vi "Dashboard Main.vi"() -> ()   [LabVIEW 2020]
uses:
  <vilib>/Utility/miscctls.llb/LVRowAndColumnTypeDef.ctl
  <vilib>/event_ctls.llb/eventvkey.ctl
  <vilib>/Rock Robotics/Network Tables/NT Read Boolean.vi
  <vilib>/Rock Robotics/WPI/Dashboard/WPI_DashboardLogging Global.vi
panel:
  in  "Camera Settings Right":T1={"Frame Rate"=30, "Compression"=30, "Size"=1, "DB Camera Config"=FALSE} {"Frame Rate" scale=1.0..30.0; "Compression" scale=100.0..-1.0; "Size" items=["640x480", "320x240", "160x120"]}
  in  "Camera Name Right":string(combo)="No Camera Selection"
  out "Camera Perf":string
  in  "Camera Settings":T1={"Frame Rate"=30, "Compression"=30, "Size"=1, "DB Camera Config"=FALSE} {"Frame Rate" scale=1.0..30.0; "Compression" scale=100.0..-1.0; "Size" items=["640x480", "320x240", "160x120"]}
  in  "TCP":refnum<k5>
  in  "Rec Mode":enum32{"Stop", "Record", "Playback"}(radio)
  out "Robot IP":string
  out "Image Message":string="Timeout in Camera Communications"
  in  "Dashboard Tab":T2(tab)
  out "Hall Effect Low":bool
  out "Limit Switch Stop":bool
  out "Elevator Encoder R":dbl
  out "Elevator Encoder L":dbl
  out "Range Detector":dbl format="%#.0f"
  out "Backwards Drive\nOn":bool
  out "Slow Speed\nOn":bool
  in  "Select Auto":string(combo)="Select Autonomous ..."
  out "NT Connection":bool
  out "Gyro":dbl(knob) scale=0.0..360.0
  out "Mode":T3(ring)=enum."Auto Disabled"
  out "Right Camera Perf":cluster{"Bandwidth (Mbps)":dbl, "FPS":dbl}
  out "Camera Image Right":T4(plugin-control)
  in  "DB/String 9":string
  in  "DB/String 8":string
  in  "DB/String 7":string
  in  "DB/String 6":string
  in  "DB/String 5":string
  in  "DB/String 4":string
  in  "DB/String 3":string
  in  "DB/String 2":string
  in  "DB/String 1":string
  in  "DB/String 0":string
  in  "DB/Slider 0":dbl(slide) scale=0.0..5.0
  in  "DB/Slider 1":dbl(slide) scale=0.0..5.0
  in  "DB/Slider 2":dbl(slide) scale=0.0..5.0
  in  "DB/Slider 3":dbl(slide) scale=0.0..5.0
  out "DB/LED 3":bool
  out "DB/LED 2":bool
  out "DB/LED 1":bool
  out "DB/LED 0":bool
  in  "DB/Button 3":bool
  in  "DB/Button 2":bool
  in  "DB/Button 1":bool
  in  "DB/Button 0":bool caption="New Name"
  in  "Test Slider":dbl(slide) scale=0.0..100.0 scale format="%#_3g"
  in  "On/Off":bool caption="Solenoid"
  in  "Test Name":u16(ring) items=["Select the test to run..."]
  in  "Test Tree":string(tree)
  in  "Motor":cluster{"Value":dbl, "Enable":bool} {"Value" scale=-1.0..1.0 scale format="%#_3g"}
  out "Progress":T5 {"Test Progress" scale=0.0..100.0}
  in  "Rev/Fwd":cluster{"Forward":bool, "Reverse":bool}
  in  "Test Ring":u16(ring) items=["Monochrome", "Color"]
  out "Cmd Status":string
  in  "Execute Command":bool
  in  "Command Params":string[][](table)
  in  "Command Selection":i32(listbox)
  in  "CheckList":i32(listbox)
  out "Tree":string(tree)
  out "Camera Image":T4(plugin-control)
  out "Background":bool
  in  "Camera Name":string(combo)="No Camera Selection"
  # "HW"
  # "HW"
  # "This tab is a great place for autonomous settings and robot-specific values.\nPlace controls and indicators inside this tab and match name to\nDashboard Variables on robot. You can also delete this comment."
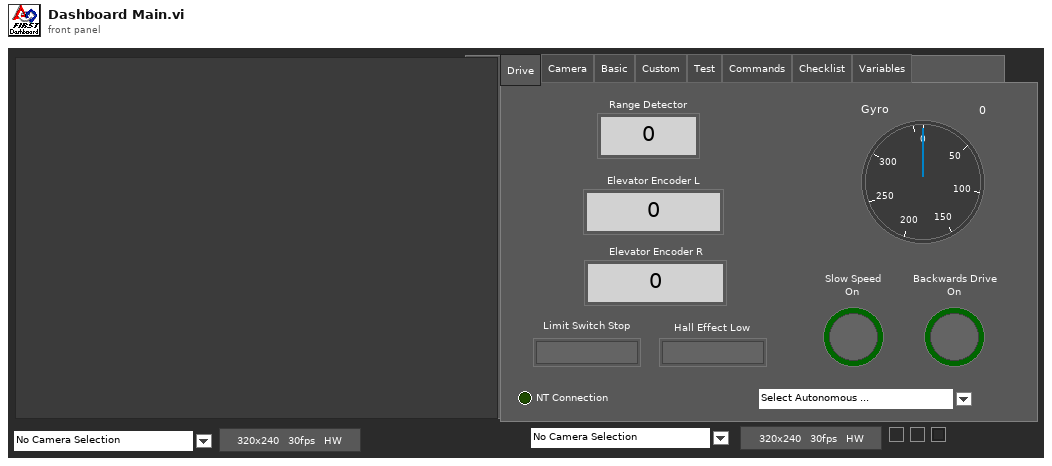
[diagram p1: front panel]
types:
  T1 = cluster{"Frame Rate":i32, "Compression":i32, "Size":u16, "DB Camera Config":bool}
  T2 = enum32{"Drive", "Camera", "Basic", "Custom", "Test", "Commands", "Checklist", "Variables"}
  T3 = enum8{"Tele-Op Disabled", "Tele-Op Enabled", "Auto Disabled", "Auto Enabled", "Test Disabled", "Test Enabled", "Disconnected", "No Code", "E-Stop"}
  T4 = typedef "IMAQ Image.ctl" = refnum<image>
  T5 = cluster{"Test Progress":u8, "Test Progress Text":string}
  T6 = cluster{"Save Path":path, "Interval (s)":dbl, "Keep":i32}
  T7 = typedef "Image Type" = u32
  T8 = cluster{"IDs":cluster{"RPC field ID":u16, "Unique ID":u16}, "String":string}
  T9 = cluster{"Error Strings":string, "Disable Counts":cluster{u16, u16}, "Rail Faults":cluster{u16, u16, u16}, "Robot IP":string, "DB Mode":u8, "Event Info":cluster{"Name":string, "Type":u8, "Number":u16, "Replay":u8}}
  T10 = cluster{"Storage":cluster{"Disk Free":u64, "RAM Block":u32, "RAM free":u32}, "CPU Utilization":cluster{"CPU % ISR":sgl, "CPU % Time Crit":sgl, "CPU % Timed Str":sgl, "CPU % High":sgl, "CPU % Above":sgl, "CPU % Normal":sgl, "CPU % Low":sgl}, "CAN":cluster{"% Bus Utilization":sgl, "Bus Off Cnt":u32, "TX_FIFO Full Cnt":u32, "Receive Error Cnt":u8, "Transmit Error Cnt":u8}, "HID":cluster{"HID Outputs":u32, "Rumble Low":u16, "Rumble High":u16}[]}
  T11 = cluster{"Status bits":cluster{"Test Mode":bool, "Autonomous":bool, "Enabled":bool, "Code Start":bool, "Brownout":bool, "Reserved 2":bool, "Reserved 3":bool, "E-Stop":bool}, "Code Trace":cluster{"Disabled":bool, "TeleOp":bool, "Auto":bool, "Test":bool}, "Controller Type":enum16{"unknown", "cRIO", "roboRio"}, "Code?":enum16{"unknown", "noCode", "code"}, "Battery V":dbl}
  T12 = cluster{"Control Bits":cluster{"TestMode":bool, "Autonomous":bool, "Enabled":bool, "FMS Present":bool, bool, bool, bool, "E-Stop":bool}, "Team Station ":u8, "Countdown":sgl, "Joystick Values":cluster{"Axes":dbl[], "Buttons":bool[], "POVs":i16[]}[]}
  T13 = cluster{"Camera Image":refnum<vi>, "Dashboard Tab":refnum<vi>, "Background":refnum<vi>, "Rec Mode":refnum<vi>, "Test Slider":refnum<vi>, "On/Off ":refnum<vi>, "Test Ring":refnum<vi>, "Rev/Fwd":refnum<vi>, "Test Name":refnum<vi>, "Motor":refnum<vi>, "Progress":refnum<vi>, "CheckList":refnum<vi>, "Tree":refnum<vi>, "Test Tree":refnum<vi>, "Command Params":refnum<vi>, "Command Selection":refnum<vi>, "Execute Command":refnum<vi>, "Cmd Status":refnum<vi>, "Camera Settings":refnum<vi>, "Camera Name":refnum<vi>, "Camera Perf":refnum<vi>, "Camera Settings Right":refnum<vi>, "Camera Name Right":refnum<vi>, "Camera Image Right":refnum<vi>}
  T14 = cluster{"Global Rectangle":i32[], "Contours":cluster{"Contour Type":u32, "ROI Type":u32, "Points":i32[]}[]}
  T15 = cluster{"Camera Name":string, string, "Saved DB Images Info":cluster{"Save Path":path, "Interval (s)":dbl, "Keep":i32}}
  T16 = cluster{"Camera Name Right":string, string, "Saved DB Images Info":cluster{"Save Path":path, "Interval (s)":dbl, "Keep":i32}}
  T17 = cluster{"Operation":enum16{"Update", "Clear"}, "Color Box":u32}[]
  T18 = typedef "eventvkey.ctl" = enum16{"ASCII", "Enter", "Return", "Shift", "Ctrl", "Alt", "Cmd", "Opt", "Caps", "NumLock", "Clear", "Break", "Up", "Down", "Left", "Right", "Insert", "Delete", "Home", "End", "PageUp", "PageDown", "Escape", "Help", "Pause", "ScrollLock", "F1", "F2", "F3", "F4", "F5", "F6", "F7", "F8", "F9", "F10", "F11", "F12", "F13", "F14", "F15", "F16", "F17", "F18", "F19", "F20", "F21", "F22", "F23", "F24", "Play", "VolumeUp", "VolumeDown", "Mute", "Two Byte Char"}
  T19 = cluster{"Image Size":bool, "Image Type":bool, "Pixel Value":bool, "ROI Information":bool, "Zoom Factor":bool}
  T20 = cluster{"Operation":enum16{"Update", "Clear"}, "Color Box":u32}
  T21 = typedef "LVRowAndColumnTypeDef.ctl" = cluster{"Row":i32, "Column":i32}
  T22 = cluster{"Shift":bool, "Ctrl":bool, "Alt":bool, "Cmd":bool, "Opt":bool}
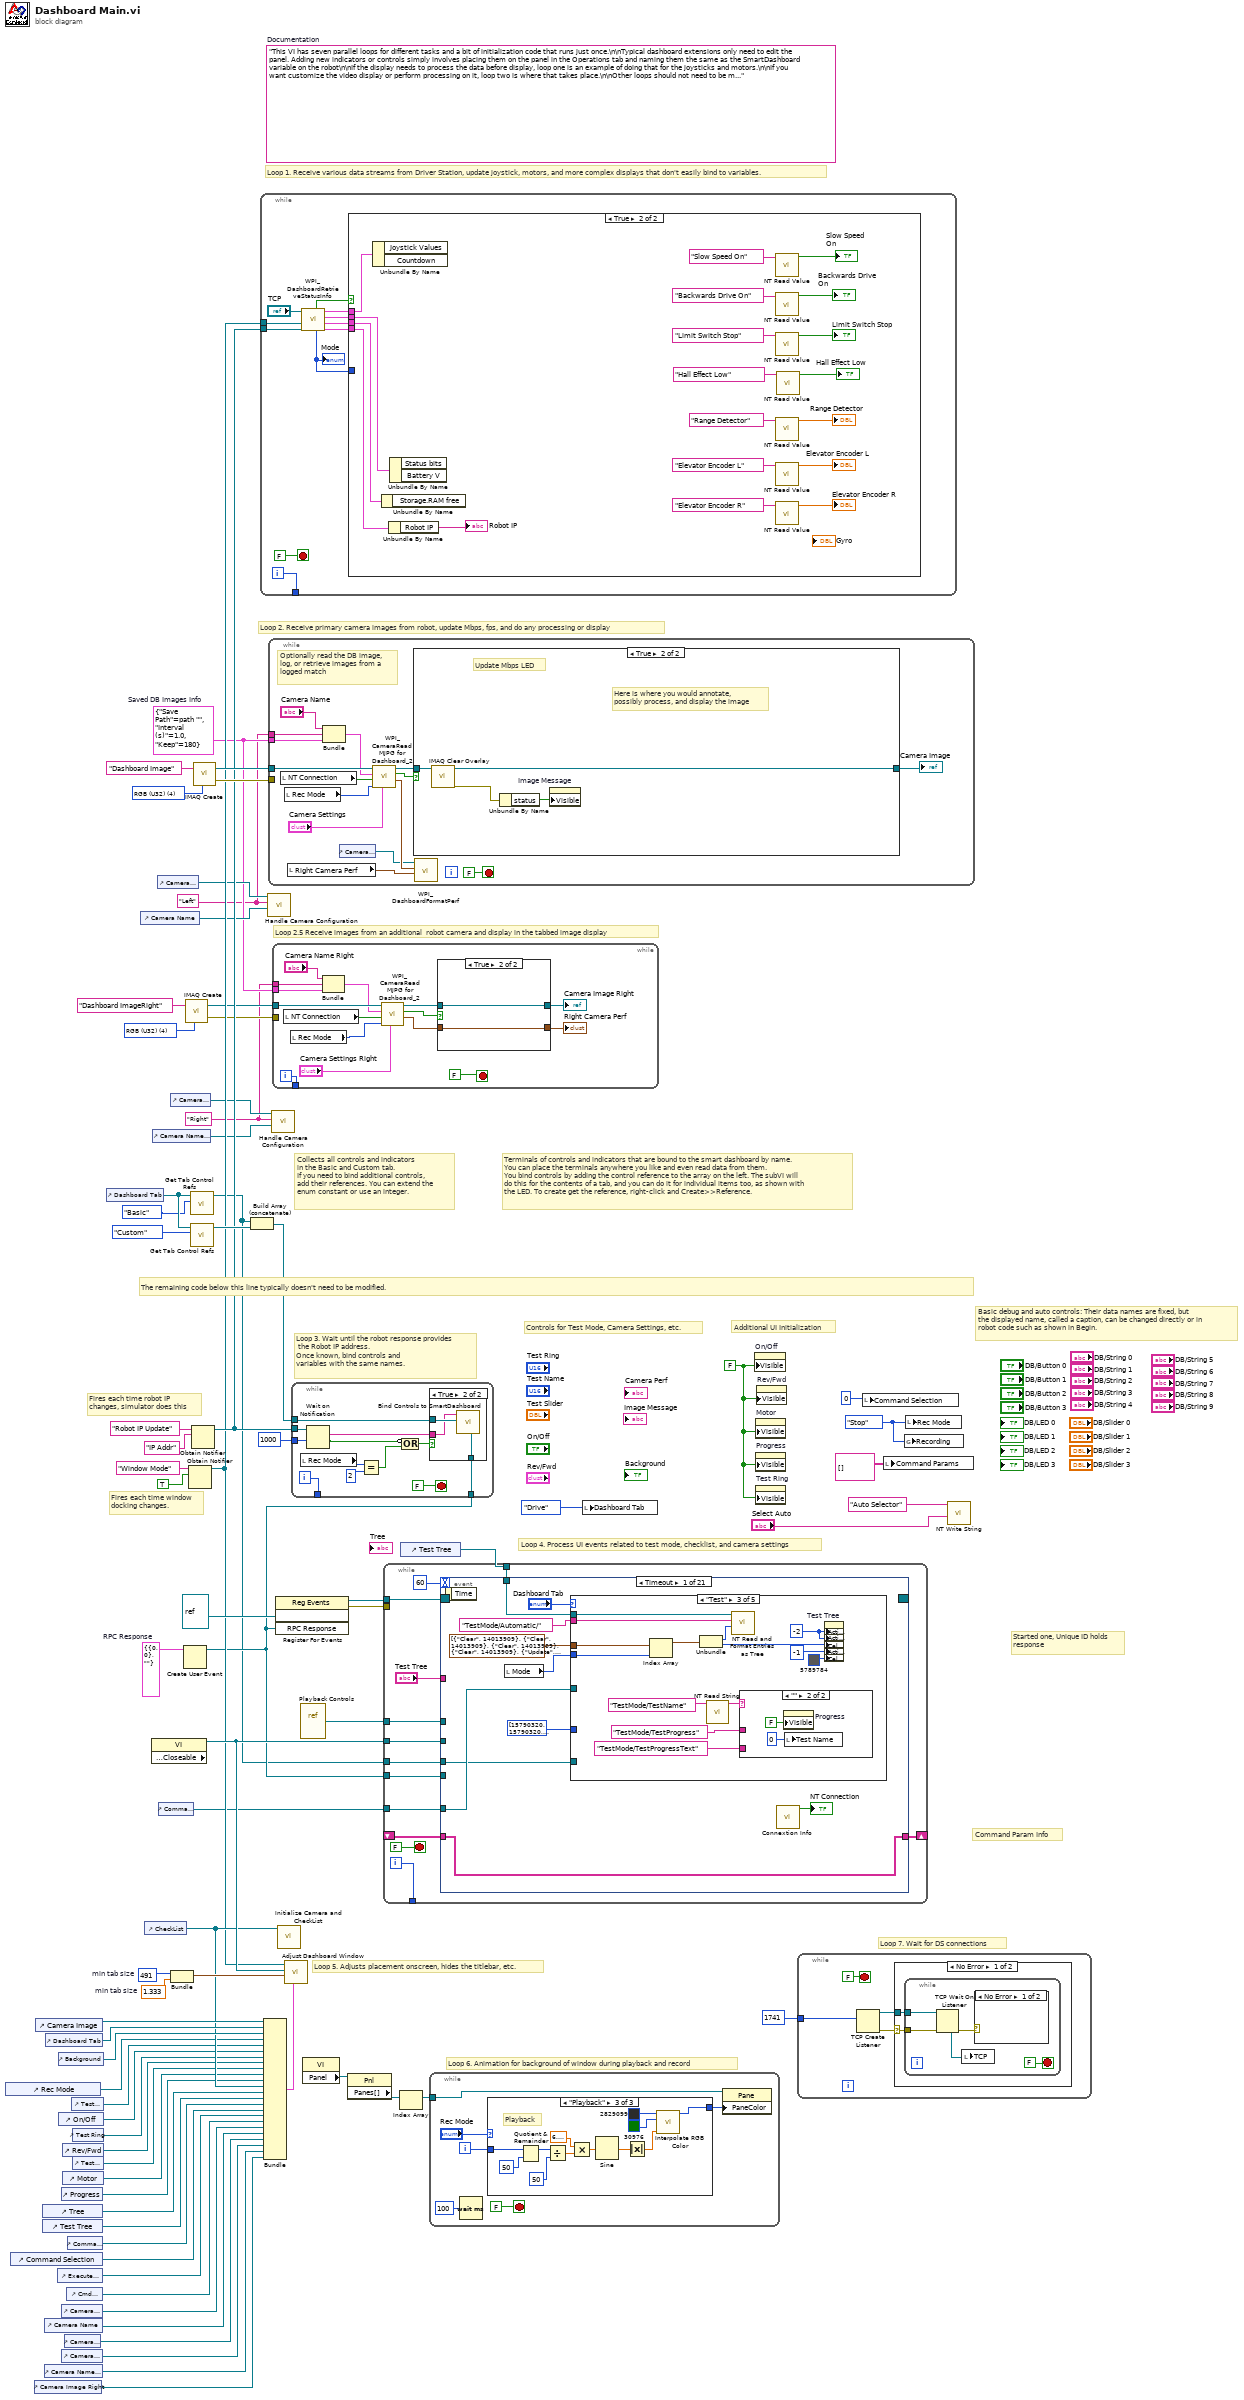
[diagram p0: block diagram]
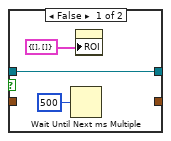
[diagram p2: hidden frame]
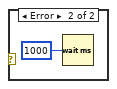
[diagram p3: hidden frame]
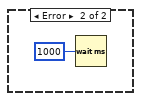
[diagram p4: hidden frame]
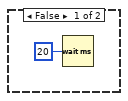
[diagram p5: hidden frame]
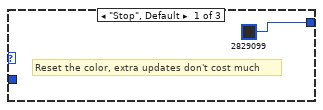
[diagram p6: hidden frame]
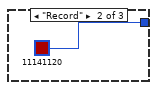
[diagram p7: hidden frame]
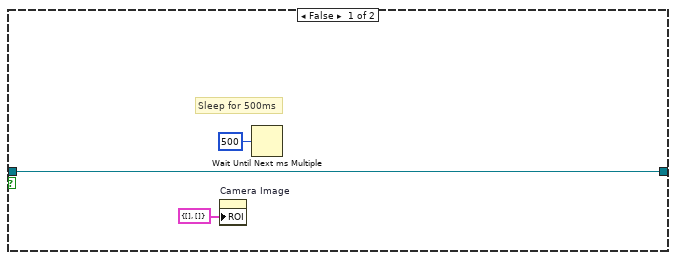
[diagram p9: hidden frame]
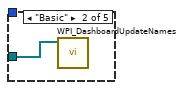
[diagram p11: hidden frame]
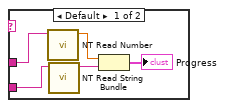
[diagram p12: hidden frame]
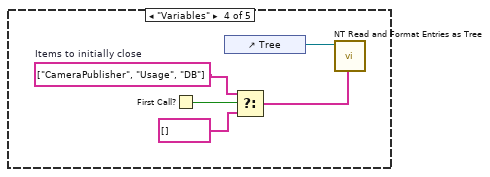
[diagram p13: hidden frame]
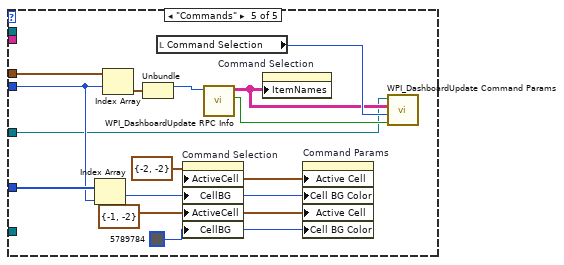
[diagram p14: hidden frame]
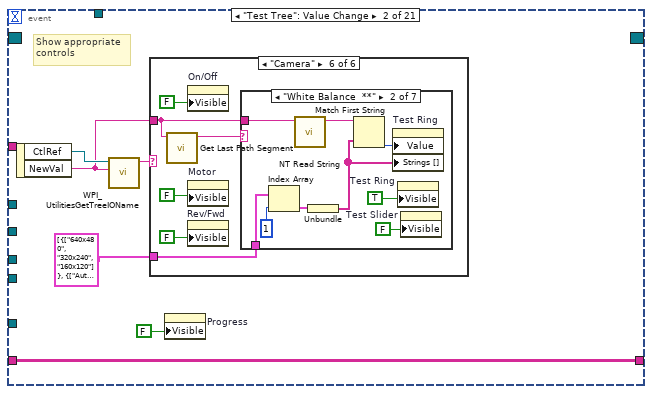
[diagram p15: hidden frame]
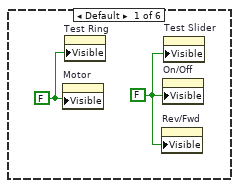
[diagram p16: hidden frame]
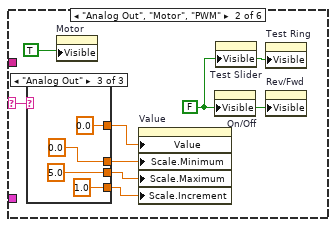
[diagram p17: hidden frame]
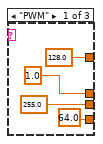
[diagram p18: hidden frame]
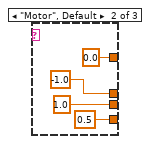
[diagram p19: hidden frame]
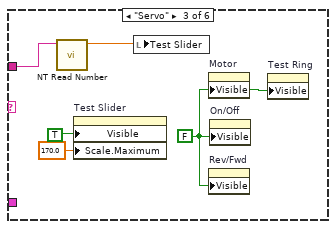
[diagram p20: hidden frame]
diagram:
  w3 = T6 {"Save Path"=path "", "Interval (s)"=1.0, "Keep"=180}  # Saved DB Images Info
  w2 = "Right"
  w1 = "Left"
  w13 = T7 4 items=["Grayscale (U8)", "Grayscale (I16)", "Grayscale (SGL)", "Complex (CSG)", "RGB (U32)", "HSL (U32)", "RGB (U64)"] ("Image Type")
  w29 = T8 {"IDs"={"RPC field ID"=0, "Unique ID"=0}, "String"=""}  # RPC Response
  w52 = 491  # min tab size
  w51 = 1.333  # min tab size
  w59 = enum32{"Stop", "Record", "Playback"}."Stop" ("Rec Mode")
  w36 = FALSE ("Visible")
  (unwired) "This VI has seven parallel loops for different tasks and a bit of initialization code that runs just once.\n\nTypical dashboard extensions only need to edit the panel. Adding new indicators or controls simply involves placing them on the panel in the Operations tab and naming them the same as the SmartDashboard variable on the robot\n\nIf the display needs to process the data before display, loop one is an example of doing that for the joysticks and motors.\n\nIf you want customize the video display or perform processing on it, loop two is where that takes place.\n\nOther loops should not need to be modified. They are pretty standard, and document the task they perform."  # Documentation
  w76 = T7 4 items=["Grayscale (U8)", "Grayscale (I16)", "Grayscale (SGL)", "Complex (CSG)", "RGB (U32)", "HSL (U32)", "RGB (U64)"] ("Image Type")
  # "Loop 2.5 Receive images from an additional  robot camera and display in the tabbed image display"
  # "Command Param Info"
  # "Started one, Unique ID holds\nresponse"
  # "Loop 7. Wait for DS connections"
  # "Basic debug and auto controls: Their data names are fixed, but\nthe displayed name, called a caption, can be changed directly or in\nrobot code such as shown in Begin."
  # "Controls for Test Mode, Camera Settings, etc."
  # "Additional UI Initialization"
  # "Loop 6. Animation for background of window during playback and record"
  # "Fires each time robot IP\nchanges, simulator does this"
  # "Fires each time window\ndocking changes."
  # "Collects all controls and indicators\nin the Basic and Custom tab.\nIf you need to bind additional controls,\nadd their references. You can extend the\nenum constant or use an integer."
  # "The remaining code below this line typically doesn't need to be modified."
  # "Loop 4. Process UI events related to test mode, checklist, and camera settings"
  # "Terminals of controls and indicators that are bound to the smart dashboard by name.\nYou can place the terminals anywhere you like and even read data from them.\nYou bind controls by adding the control reference to the array on the left. The subVI will\ndo this for the contents of a tab, and you can do it for individual items too, as shown with\nthe LED. To create get the reference, right-click and Create>>Reference."
  # "Loop 3. Wait until the robot response provides\n the Robot IP address.\nOnce known, bind controls and\nvariables with the same names."
  # "Loop 5. Adjusts placement onscreen, hides the titlebar, etc."
  # "Loop 1. Receive various data streams from Driver Station, update joystick, motors, and more complex displays that don't easily bind to variables."
  # "Loop 2. Receive primary camera images from robot, update Mbps, fps, and do any processing or display"
  n1 = control-ref of="Rec Mode"() -> (w42:refnum<vi>)
  n2 = control-ref of="Command Selection"() -> (w28:refnum<vi>)
  n3 = control-ref of="Camera Image Right"() -> (w6:refnum<vi>)
  n4 = control-ref of="Camera Image"() -> (w54:refnum<vi>)
  n5 = control-ref of="Tree"() -> (w46:refnum<vi>)
  n6 = control-ref of="Test Tree"() -> (w45:refnum<vi>)
  n7 = control-ref of="Camera Name"() -> (w19:refnum<vi>)
  n8 = control-ref of="Camera Name Right"() -> (w7:refnum<vi>)
  n9 = control-ref of="Dashboard Tab"() -> (w53:refnum<vi>)
  n10 = control-ref of="Execute Command"() -> (w30:refnum<vi>)
  n11 = control-ref of="Background"() -> (w49:refnum<vi>)
  n12 = control-ref of="On/Off"() -> (w40:refnum<vi>)
  n13 = control-ref of="Progress"() -> (w37:refnum<vi>)
  n14 = control-ref of="Camera Settings"() -> (w20:refnum<vi>)
  n15 = control-ref of="Camera Settings Right"() -> (w8:refnum<vi>)
  n16 = control-ref of="Rev/Fwd"() -> (w38:refnum<vi>)
  n17 = control-ref of="Motor"() -> (w43:refnum<vi>)
  n18 = control-ref of="Camera Perf"() -> (w18:refnum<vi>)
  n19 = control-ref of="Cmd Status"() -> (w24:refnum<vi>)
  n20 = control-ref of="Command Params"() -> (w31:refnum<vi>)
  n21 = control-ref of="Test Slider"() -> (w41:refnum<vi>)
  n22 = control-ref of="Test Ring"() -> (w39:refnum<vi>)
  n23 = control-ref of="Test Name"() -> (w44:refnum<vi>)
  n24 = control-ref of="Dashboard Tab"() -> (w57:refnum<vi>)
  n25 = control-ref of="Camera Name"() -> (w21:refnum<vi>)
  n26 = control-ref of="CheckList"() -> (w47:refnum<vi>)
  n27 = property class="VI" props=["Front Panel.Closeable"]() -> (reference out=w58:refnum<vi>)  [unwired: 2 in, 2 out]
  n28 = control-ref of="Camera Name Right"() -> (w9:refnum<vi>)
  n29 = control-ref of="Camera Settings"() -> (w22:refnum<vi>)
  n30 = control-ref of="Command Params"() -> (w23:refnum<vi>)
  n31 = control-ref of="Camera Settings Right"() -> (w10:refnum<vi>)
  n32 = Bundle("min tab size"=w52, "min tab size"=w51) -> (w50:cluster{"min tab size":i32, "min tab size":dbl})  [unwired: 1 in]
  n33 = Create User Event(user event datatype=w29) -> (user event=w25:refnum<user-event>)  [unwired: 1 in, 1 out]
  n34 = call "IMAQ Create"("Image Name"="Dashboard ImageRight", "Image Type"=w13) -> ("New Image"=w12:T4, "error out"=w11:errorcluster)  [unwired: 2 in, 1 out]
  n35 = Obtain Notifier(name (unnamed)="Window Mode", notification data type=TRUE) -> (notifier out=w34:refnum<notifier>)  [unwired: 2 in, 2 out]
  n36 = call <vilib>:"Get Tab Control Refs.vi"("Page Index"=T2."Basic" ("Dashboard Tab"), "TabControl in"=w57) -> ("ControlsOnPage"=w17:refnum<vi>[])  [unwired: 9 in]
  n37 = call <vilib>:"Get Tab Control Refs.vi"("Page Index"=T2."Custom" ("Dashboard Tab"), "TabControl in"=w57) -> ("ControlsOnPage"=w56:refnum<vi>[])  [unwired: 9 in]
  n38 = Obtain Notifier(name (unnamed)="Robot IP Update", notification data type="IP Addr" ("name (unnamed)")) -> (notifier out=w35:refnum<notifier>)  [unwired: 2 in, 2 out]
  n39 = call "IMAQ Create"("Image Name"="Dashboard Image", "Image Type"=w76) -> ("New Image"=w74:T4, "error out"=w73:errorcluster)  [unwired: 2 in, 1 out]
  n40 = Build Array (concatenate)(w17, w56) -> (w55:refnum<vi>[])
  n41 = while {
    tunnel: [w86] -> _
    tunnel: w35 -> [w80]
    tunnel: w34 -> [w77]
    i -> [w86]
    stop <- FALSE stop-if-true
    n42 = call <vilib>:"WPI_DashboardRetrieveStatusInfo.vi"("Binding Refnum"=w80, "Window Mode Notifier"=w77, "TCP Cnx"="TCP") -> ("Power and Errors"=w81:T9, "Robot Metrics"=w84:T10, "Status Info"=w85:T11, "Control Info"=w82:T12, "Robot Mode"=w79:T3, "Process?"=w83:bool)  [unwired: 3 in]
    "Mode" <- w79
    n43 = case shown="True" w83 {
      tunnel: w85 -> [_ w107]
      tunnel: w84 -> [_ w106]
      tunnel: w82 -> [_ w105]
      tunnel: w81 -> [_ w104]
      tunnel: w79 -> [_ _]
      frame False {
        n44 = Wait (ms)(milliseconds to wait=u32 20) -> ()  [unwired: 1 out]
      }
      frame True {
        n45 = Unbundle By Name(w105) -> ()  [unwired: 2 out]
        n46 = Unbundle By Name(w106) -> ()  [unwired: 1 out]
        n47 = Unbundle By Name(w104) -> ("Robot IP"=→"Robot IP":string)
        n48 = Unbundle By Name(w107) -> ()  [unwired: 2 out]
        n49 = call-poly <vilib>:"NT Read Value.vi"("Name"="Slow Speed On") -> ("Boolean"=→"Slow Speed\nOn":bool)  [unwired: 9 in, 1 out]
        n50 = call-poly <vilib>:"NT Read Value.vi"("Name"="Backwards Drive On") -> ("Boolean"=→"Backwards Drive\nOn":bool)  [unwired: 9 in, 1 out]
        n51 = call-poly <vilib>:"NT Read Value.vi"("Name"="Limit Switch Stop") -> ("Boolean"=→"Limit Switch Stop":bool)  [unwired: 9 in, 1 out]
        n52 = call-poly <vilib>:"NT Read Value.vi"("Name"="Range Detector") -> ("Numeric"=→"Range Detector":dbl)  [unwired: 9 in, 1 out]
        n53 = call-poly <vilib>:"NT Read Value.vi"("Name"="Elevator Encoder L") -> ("Numeric"=→"Elevator Encoder L":dbl)  [unwired: 9 in, 1 out]
        n54 = call-poly <vilib>:"NT Read Value.vi"("Name"="Elevator Encoder R") -> ("Numeric"=→"Elevator Encoder R":dbl)  [unwired: 9 in, 1 out]
        n55 = call-poly <vilib>:"NT Read Value.vi"("Name"="Hall Effect Low") -> ("Boolean"=→"Hall Effect Low":bool)  [unwired: 9 in, 1 out]
      }
    }
  }
  n56 = Bundle("Camera Image"=w54, "Dashboard Tab"=w53, "Background"=w49, "Rec Mode"=w42, "Test Slider"=w41, "On/Off"=w40, "Test Ring"=w39, "Rev/Fwd"=w38, "Test Name"=w44, "Motor"=w43, "Progress"=w37, "CheckList"=w47, "Tree"=w46, "Test Tree"=w45, "Command Params"=w31, "Command Selection"=w28, "Execute Command"=w30, "Cmd Status"=w24, "Camera Settings"=w20, "Camera Name"=w19, "Camera Perf"=w18, "Camera Settings Right"=w8, "Camera Name Right"=w7, "Camera Image Right"=w6) -> (w48:T13)  [unwired: 1 in]
  n57 = call "Handle Camera Configuration.vi"("CameraNameRef"=w21, "Display Name"=w1, "ClusterRef"=w22) -> ()  [unwired: 9 in]
  n58 = while {
    tunnel: w74 -> [w121]
    tunnel: w73 -> [_]
    tunnel: w3 -> [w114]
    tunnel: w1 -> [w111]
    stop <- FALSE stop-if-true
    # "Optionally read the DB image,\nlog, or retrieve images from a\nlogged match"
    n59 = local read "NT Connection"() -> (w115:bool)
    n60 = local read "Rec Mode"() -> (w118:enum32{"Stop", "Record", "Playback"})
    n61 = local read "Right Camera Perf"() -> (w109:cluster{"Bandwidth (Mbps)":dbl, "FPS":dbl})
    n62 = Bundle("Camera Name"="Camera Name", w111, "Saved DB Images Info"=w114) -> (w113:T15)  [unwired: 1 in]
    n63 = control-ref of="Camera Perf"() -> (w108:refnum<vi>)
    n64 = call <vilib>:"WPI_CameraRead MJPG for Dashboard_2.vi"("Camera Settings"="Camera Settings", "Rec Mode"=w118, "NT Connection"=w115, "Capture Info"=w113, "Image in"=w121) -> ("perf info"=w110:cluster{"Bandwidth (Mbps)":dbl, "fps":dbl}, "Active"=w119:bool, "Image\\ out"=w120:T4)  [unwired: 4 in]
    n65 = case shown="True" w119 {
      tunnel: w120 -> [w124 w127]
      tunnel: [w124 w126] -> w116
      frame False {
        # "Sleep for 500ms"
        n66 = property on="Camera Image" class="ImageControl"("ROI"=T14 {"Global Rectangle"=[], "Contours"=[]}) -> ()  [unwired: 2 in, 2 out]
        n67 = Wait Until Next ms Multiple(millisecond multiple=u32 500) -> ()  [unwired: 1 out]
      }
      frame True {
        # "Here is where you would annotate,\npossibly process, and display the image"
        # "Update Mbps LED"
        n68 = call "IMAQ Clear Overlay"("Image"=w127) -> ("error out"=w128:errorcluster, "Image Out"=w126:T4)  [unwired: 2 in, 7 out]
        n69 = Unbundle By Name(w128) -> ("status"=w129:bool)
        n70 = property on="Image Message" class="Str"("Visible"=w129) -> ()  [unwired: 2 in, 2 out]
      }
    }
    "Camera Image" <- w116
    n71 = call <vilib>:"WPI_DashboardFormatPerf.vi"("Right Camera Perf"=w109, "Performance"=w110, "String in"=w108) -> ()  [unwired: 9 in]
  }
  n72 = call "Handle Camera Configuration.vi"("CameraNameRef"=w9, "Display Name"=w2, "ClusterRef"=w10) -> ()  [unwired: 9 in]
  n73 = while {
    tunnel: w12 -> [w144]
    tunnel: w11 -> [_]
    tunnel: [w139] -> _
    tunnel: w3 -> [w135]
    tunnel: w2 -> [w132]
    i -> [w139]
    stop <- FALSE stop-if-true
    n74 = local read "NT Connection"() -> (w136:bool)
    n75 = local read "Rec Mode"() -> (w143:enum32{"Stop", "Record", "Playback"})
    n76 = Bundle("Camera Name Right"="Camera Name Right", w132, "Saved DB Images Info"=w135) -> (w134:T16)  [unwired: 1 in]
    n77 = call <vilib>:"WPI_CameraRead MJPG for Dashboard_2.vi"("Camera Settings"="Camera Settings Right", "Rec Mode"=w143, "NT Connection"=w136, "Capture Info"=w134, "Image in"=w144) -> ("perf info"=w130:cluster{"Bandwidth (Mbps)":dbl, "fps":dbl}, "Active"=w138:bool, "Image\\ out"=w141:T4)  [unwired: 4 in]
    n78 = case shown="True" w138 {
      tunnel: w141 -> [w146 w149]
      tunnel: [w146 w149] -> w137
      tunnel: [_ w148] -> w131
      tunnel: w130 -> [_ w148]
      frame False {
        n79 = Wait Until Next ms Multiple(millisecond multiple=u32 500) -> ()  [unwired: 1 out]
        n80 = property on="Camera Image Right" class="ImageControl"("ROI"=T14 {"Global Rectangle"=[], "Contours"=[]}) -> ()  [unwired: 2 in, 2 out]
      }
      frame True {
      }
    }
    "Camera Image Right" <- w137
    "Right Camera Perf" <- w131
  }
  n81 = register-events(refnum<vi> refnum, w25) -> (reference out=w63:refnum<event-registration>, error out=w62:errorcluster)  [unwired: 2 in]
  n82 = call "Initialize Camera and CheckList.vi"("ListBox in"=w47) -> ()  [unwired: 11 in]
  n83 = call "Adjust Dashboard Window.vi"("Sizing Refnums"=w48, "Size Constraints"=w50, "VI"=w58, "WIn Mode"=w34) -> ()  [unwired: 8 in]
  n84 = while {
    tunnel: w55 -> [w161]
    tunnel: w35 -> [w159]
    tunnel: [w157] -> _
    tunnel: u32 1000 ("milliseconds to wait") -> [w156]
    tunnel: w25 -> [w150]
    i -> [w157]
    stop <- FALSE stop-if-true
    n85 = local read "Rec Mode"() -> (w152:enum32{"Stop", "Record", "Playback"})
    n86 = Wait on Notification(notifier=w159, timeout in ms (-1)=w156) -> (notification=w158:string, timed out?=w154:bool)  [unwired: 2 in, 2 out]
    n87 = Equal?(x=w152, y=u16 2 ("Rec Mode")) -> (x = y?=w153:bool)
    n88 = Compound Arithmetic op=OR(invert w154, w153) -> (w155:bool)
    n89 = case shown="True" w155 {
      tunnel: w161 -> [_ w164]
      tunnel: w158 -> [_ w163]
      tunnel: w150 -> [_ w162]
      frame False {
      }
      frame True {
        n90 = call <vilib>:"Bind Controls to SmartDashboard.vi"("RPC ref"=w162, "Bound Control Refs"=w164, "Server IP Address"=w163) -> ()  [unwired: 9 in]
      }
    }
  }
  n91 = vi-ref "Playback Controls.vi"() -> (w64:refnum<vi>)
  n92 = property class="VI"() -> ("Panel"=w66:refnum<vi>)  [unwired: 2 in, 2 out]
  n93 = property class="Pnl"(reference=w66) -> ("Panes[]"=w67:refnum<vi>[])  [unwired: 1 in, 2 out]
  n94 = Index Array(array=w67) -> (element=w65:refnum<vi>)  [unwired: 1 in]
  n95 = control-ref of="Test Tree"() -> (w68:refnum<vi>)
  n96 = while {
    tunnel: [w174] -> _
    tunnel: w68 -> [w173]
    tunnel: w64 -> [w172]
    tunnel: w63 -> [w171]
    tunnel: w62 -> [_]
    tunnel: w58 -> [w170]
    tunnel: w25 -> [w169]
    tunnel: w23 -> [w168]
    shift-right: [w167] -> _
    shift-left: _ -> [w166]
    tunnel: w17 -> [w165]
    i -> [w174]
    stop <- FALSE stop-if-true
    n97 = event shown="[0] Timeout" {
      selector: w171 -> [_ _ _ _ _ _ _ _ _ _ _ _ _ _ _ _ _ _ _ _ _]
      dyn-events: [_ _ _ _ _ _ _ _ _ _ _ _ _ _ _ _ w434 _ _ _ _] -> _
      timeout: u32 60 ("milliseconds to wait") -> [_ _ _ _ _ _ _ _ _ _ _ _ _ _ _ _ _ _ _ _ _]
      tunnel: w173 -> [w186 _ _ _ _ _ _ _ _ _ _ _ _ _ _ _ _ _ _ _ _]
      tunnel: "Test Tree" -> [_ _ _ _ _ _ _ _ _ _ _ w401 w409 w411 w415 w423 _ _ _ _ _]
      tunnel: w172 -> [_ _ _ _ _ _ _ _ _ _ _ _ _ _ _ _ w436 _ w454 _ _]
      tunnel: w170 -> [_ _ _ _ _ _ _ _ _ _ _ _ _ _ _ _ w432 _ _ _ _]
      tunnel: w169 -> [_ _ _ _ _ _ _ _ _ _ _ _ _ _ _ _ w430 _ _ _ _]
      tunnel: w168 -> [w181 _ _ _ _ _ w352 _ _ _ _ _ _ _ _ _ _ _ _ _ _]
      tunnel: [w180 w229 w331 w336 w345 w349 w350 w359 w369 w376 w388 w400 w407 w410 w414 w422 w429 w449 w451 w455 w468] -> w167
      tunnel: w166 -> [w180 w229 w331 w336 w345 w349 w350 _ _ w376 w388 w400 w407 w410 w414 w422 w429 w449 w451 w455 w468]
      tunnel: w165 -> [w178 _ _ _ _ _ _ _ _ _ _ _ _ _ _ _ _ _ _ _ _]
      event Timeout {
        n98 = event-data() -> ()  [unwired: 1 in, 1 out]
        n99 = local read "Mode"() -> (w183:T3)
        n100 = case shown="\"Test\"" "Dashboard Tab" {
          tunnel: w186 -> [_ _ w202 _ _]
          tunnel: "TestMode/Automatic/" ("Name Pattern") -> [_ _ w201 _ _]
          tunnel: T17 [{"Operation"=enum."Clear", "Color Box"=14013909}, {"Operation"=enum."Clear", "Color Box"=14013909}, {"Operation"=enum."Clear", "Color Box"=14013909}, {"Operation"=enum."Clear", "Color Box"=14013909}, {"Operation"=enum."Update", "Color Box"=14013909}, {"Operation"=enum."Update", "Color Box"=16777215}, {"Operation"=enum."Clear", "Color Box"=14013909}, {"Operation"=enum."Clear", "Color Box"=14013909}, {"Operation"=enum."Clear", "Color Box"=14013909}] -> [_ _ w194 _ w222]
          tunnel: w183 -> [_ _ w193 _ w221]
          tunnel: u32[] [15790320, 15790320, 15790320, 15790320, 16777215, 16777215, 15790320, 15790320, 15790320] -> [_ _ _ _ w227]
          tunnel: w181 -> [_ _ _ _ w215]
          tunnel: w178 -> [_ w188 _ _ _]
          frame "Custom", Default {
          }
          frame "Basic" {
            n101 = call <vilib>:"WPI_DashboardUpdateNames.vi"("Controls on Tab"=w188) -> ()  [unwired: 11 in]
          }
          frame "Test" {
            w200 = -2 ("Active Item:Row Number")
            n102 = Index Array(array=w194, index=w193) -> (element=w195:T20)
            n103 = Unbundle(w195) -> ("Operation"=w196:enum16{"Update", "Clear"}, "Color Box"=w197:u32)
            n104 = call <vilib>:"NT Read String.vi"("Name"="TestMode/TestName") -> ("String"=w191:string)  [unwired: 9 in, 1 out]
            n105 = call <vilib>:"NT Read and Format Entries as Tree.vi"("Operation"=w196, "Name Pattern"=w201, "Tree Refnum"=w202) -> ()  [unwired: 7 in, 2 out]
            n106 = case shown="\"\"" w191 {
              tunnel: "TestMode/TestProgress" ("Name") -> [w204 _]
              tunnel: "TestMode/TestProgressText" ("Name") -> [w203 _]
              frame Default {
                n107 = call <vilib>:"NT Read Number.vi"("Name"=w204) -> ("Numeric"=w205:dbl)  [unwired: 9 in, 1 out]
                n108 = call <vilib>:"NT Read String.vi"("Name"=w203) -> ("String"=w206:string)  [unwired: 9 in, 1 out]
                n109 = Bundle("Numeric"=w205, "String"=w206) -> (→"Progress":cluster{"Numeric":dbl, "String":string})  [unwired: 1 in]
              }
              frame "" {
                n110 = property on="Progress" class="Clust (strict)"("Visible"=FALSE) -> ()  [unwired: 2 in, 2 out]
                n111 = local write "Test Name"(u16 0) -> ()
              }
            }
            n112 = property on="Test Tree" class="Tree (strict)"("Active Item Row Number"=w200, "ActiveColNum"=w200, "CellBG"=w197, "Active Item Row Number"=-1 ("Active Item:Row Number"), "CellBG"=u32 5789784 ("Color Box")) -> ()  [unwired: 2 in, 2 out]
          }
          frame "Variables" {
            w212 = string[] ["CameraPublisher", "Usage", "DB"]  # Items to initially close
            n113 = First Call?() -> (First Call?: T/F=w213:bool)
            n114 = control-ref of="Tree"() -> (w214:refnum<vi>)
            n115 = Select(t=w212, s=w213, f=string[] []) -> (s? t:f=w210:string[])
            n116 = call <vilib>:"NT Read and Format Entries as Tree.vi"("Tags to  Close"=w210, "Tree Refnum"=w214) -> ()  [unwired: 8 in, 2 out]
          }
          frame "Commands" {
            w223 = u32 5789784 ("Color Box")
            w224 = T21 {"Row"=-1, "Column"=-2} ("Active Cell:Active Cell")
            w226 = T21 {"Row"=-2, "Column"=-2} ("Active Cell:Active Cell")
            n117 = Index Array(array=w227, index=w221) -> (element=w225:u32)
            n118 = Index Array(array=w222, index=w221) -> (element=w220:T20)
            n119 = Unbundle(w220) -> ("Operation"=w219:enum16{"Update", "Clear"})  [unwired: 1 out]
            n120 = local read "Command Selection"() -> (w218:i32)
            n121 = property on="Command Selection" class="MCListbox (strict)"("ActiveCell"=w226, "CellBG"=w225, "ActiveCell"=w224, "CellBG"=w223) -> ()  [unwired: 2 in, 2 out]
            n122 = call <vilib>:"WPI_DashboardUpdate RPC Info.vi"("Operation"=w219) -> ("update"=w217:bool, "commands"=w216:string[][])  [unwired: 9 in]
            n123 = property on="Command Selection" class="MCListbox (strict)"("ItemNames"=w216) -> ()  [unwired: 2 in, 2 out]
            n124 = property on="Command Params" class="Tbl (strict)"("Active Cell"=w226, "Cell BG Color"=w225, "Active Cell"=w224, "Cell BG Color"=w223) -> ()  [unwired: 2 in, 2 out]
            n125 = call <vilib>:"WPI_DashboardUpdate Command Params.vi"("Update"=w217, "NewVal"=w218, "Commands"=w216, "Param Tbl"=w215) -> ()  [unwired: 7 in, 1 out]
          }
        }
        n126 = call <vilib>:"Connextion Info.vi"() -> ("Connected"=→"NT Connection":bool)  [unwired: 10 in, 1 out]
      }
      event "Test Tree": Value Change {
        # "Show appropriate\ncontrols"
        n127 = event-data() -> ("CtlRef"=w232:refnum<vi>, "NewVal"=w230:string)  [unwired: 1 in]
        n128 = call <vilib>:"WPI_UtilitiesGetTreeIOName.vi"("NewVal"=w230, "TreeControl in"=w232) -> ("I/O Name"=w233:string)  [unwired: 9 in]
        n129 = case shown="\"Camera\"" w233 {
          selector: w233 -> [_ w240 _ w262 w271 _]
          tunnel: w230 -> [_ _ w259 w261 _ w278]
          tunnel: cluster{string[]}[] [{["640x480", "320x240", "160x120"]}, {["Auto", "Fixed indoor", "Fixed outdoor 1", "Fixed outdoor 2", "Fixed fluorescent 1", "Fixed fluorescent 2", "Hold current"]}, {["Auto", "Flicker-free 50 Hz", "Flicker-free 60 Hz", "Hold current"]}, {["None", "Prioritize frame rate", "Prioritize image quality"]}, {["Monochrome", "Color"]}] -> [_ _ _ _ _ w277]
          frame Default {
            w235 = FALSE ("Visible")
            w234 = FALSE ("Visible")
            n130 = property on="Motor" class="Clust (strict)"("Visible"=w234) -> ()  [unwired: 2 in, 2 out]
            n131 = property on="Test Ring" class="Ring (strict)"("Visible"=w234) -> ()  [unwired: 2 in, 2 out]
            n132 = property on="Rev/Fwd" class="Clust (strict)"("Visible"=w235) -> ()  [unwired: 2 in, 2 out]
            n133 = property on="On/Off" class="Bool (strict)"("Visible"=w235) -> ()  [unwired: 2 in, 2 out]
            n134 = property on="Test Slider" class="Slide (strict)"("Visible"=w235) -> ()  [unwired: 2 in, 2 out]
          }
          frame "Analog Out", "Motor", "PWM" {
            w241 = FALSE ("Visible")
            n135 = case shown="\"Analog Out\"" w240 {
              tunnel: [1.0 ("Value") -1.0 ("Value") 0.0 ("Value")] -> w239
              tunnel: [255.0 ("Value") 1.0 ("Value") 5.0 ("Value")] -> w238
              tunnel: [128.0 ("Value") 0.0 ("Value") 0.0 ("Value")] -> w237
              tunnel: [64.0 ("Value") 0.5 ("Value") 1.0 ("Value")] -> w236
              frame "PWM" {
              }
              frame "Motor", Default {
              }
              frame "Analog Out" {
              }
            }
            n136 = property on="Motor" class="Clust (strict)"("Visible"=TRUE) -> ()  [unwired: 2 in, 2 out]
            n137 = property on="Value" class="Slide (strict)"("Value"=w237, "Scale.Minimum"=w239, "Scale.Maximum"=w238, "Scale.Increment"=w236) -> ()  [unwired: 2 in, 2 out]
            n138 = property on="On/Off" class="Bool (strict)"("Visible"=w241) -> ()  [unwired: 2 in, 2 out]
            n139 = property on="Test Slider" class="Slide (strict)"("Visible"=w241) -> ()  [unwired: 2 in, 2 out]
            n140 = property on="Test Ring" class="Ring (strict)"("Visible"=w241) -> ()  [unwired: 2 in, 2 out]
            n141 = property on="Rev/Fwd" class="Clust (strict)"("Visible"=w241) -> ()  [unwired: 2 in, 2 out]
          }
          frame "Servo" {
            w257 = FALSE ("Visible")
            n142 = call <vilib>:"NT Read Number.vi"("Name"=w259) -> ("Numeric"=w258:dbl)  [unwired: 9 in, 1 out]
            n143 = property on="Test Slider" class="Slide (strict)"("Visible"=TRUE, "Scale.Maximum"=170.0 ("Scale.Range:Maximum")) -> ()  [unwired: 2 in, 2 out]
            n144 = local write "Test Slider"(w258) -> ()
            n145 = property on="Motor" class="Clust (strict)"("Visible"=w257) -> ()  [unwired: 2 in, 2 out]
            n146 = property on="Rev/Fwd" class="Clust (strict)"("Visible"=w257) -> ()  [unwired: 2 in, 2 out]
            n147 = property on="On/Off" class="Bool (strict)"("Visible"=w257) -> ()  [unwired: 2 in, 2 out]
            n148 = property on="Test Ring" class="Ring (strict)"("Visible"=w257) -> ()  [unwired: 2 in, 2 out]
          }
          frame "Relay", "Solenoid" {
            w260 = FALSE ("Visible")
            n149 = property on="Motor" class="Clust (strict)"("Visible"=w260) -> ()  [unwired: 2 in, 2 out]
            n150 = property on="Test Slider" class="Slide (strict)"("Visible"=w260) -> ()  [unwired: 2 in, 2 out]
            n151 = Search and Replace String(input string=w261, search string="/Value  **", replace string="/Direction") -> (result string=w267:string)  [unwired: 5 in, 3 out]
            n152 = property on="Test Ring" class="Ring (strict)"("Visible"=w260) -> ()  [unwired: 2 in, 2 out]
            n153 = call <vilib>:"NT Read String.vi"("Name"=w267) -> ("String"=w265:string)  [unwired: 9 in, 1 out]
            n154 = Equal?(x="Both directions", y=w265) -> (x = y?=w263:bool)
            n155 = Not(x=w263) -> (.not. x?=w264:bool)
            n156 = property on="Rev/Fwd" class="Clust (strict)"("Visible"=w263) -> ()  [unwired: 2 in, 2 out]
            n157 = property on="On/Off" class="Bool (strict)"("Visible"=w264, "Caption.Text"=w262) -> ()  [unwired: 2 in, 2 out]
          }
          frame "Compressor", "Digital Out" {
            w270 = FALSE ("Visible")
            # "Get direction and finish"
            n158 = property on="Motor" class="Clust (strict)"("Visible"=w270) -> ()  [unwired: 2 in, 2 out]
            n159 = property on="Test Slider" class="Slide (strict)"("Visible"=w270) -> ()  [unwired: 2 in, 2 out]
            n160 = property on="Test Ring" class="Ring (strict)"("Visible"=w270) -> ()  [unwired: 2 in, 2 out]
            n161 = property on="On/Off" class="Bool (strict)"("Visible"=TRUE, "Caption.Text"=w271) -> ()  [unwired: 2 in, 2 out]
            n162 = property on="Rev/Fwd" class="Clust (strict)"("Visible"=FALSE) -> ()  [unwired: 2 in, 2 out]
          }
          frame "Camera" {
            n163 = call <vilib>:"Get Last Path Segment.vi"("String in"=w278) -> ("String out"=w279:string)  [unwired: 10 in]
            n164 = property on="On/Off" class="Bool (strict)"("Visible"=FALSE) -> ()  [unwired: 2 in, 2 out]
            n165 = property on="Motor" class="Clust (strict)"("Visible"=FALSE) -> ()  [unwired: 2 in, 2 out]
            n166 = property on="Rev/Fwd" class="Clust (strict)"("Visible"=FALSE) -> ()  [unwired: 2 in, 2 out]
            n167 = case shown="\"White Balance  **\"" w279 {
              tunnel: w278 -> [w285 w294 w303 w312 w321 _ w327]
              tunnel: w277 -> [w283 w291 w300 w309 w318 _ _]
              frame "Size  **" {
                n168 = Index Array(array=w283) -> (element=w282:cluster{string[]})  [unwired: 1 in]
                n169 = call <vilib>:"NT Read String.vi"("Name"=w285) -> ("String"=w284:string)  [unwired: 9 in, 1 out]
                n170 = Unbundle(w282) -> (w280:string[])
                n171 = Match First String(2:w280, 3:w284) -> (0:w281:i32)  [unwired: 1 out]
                n172 = property on="Test Ring" class="Ring (strict)"("Value"=w281, "Strings []"=w280) -> ()  [unwired: 2 in, 2 out]
                n173 = property on="Test Ring" class="Ring (strict)"("Visible"=TRUE) -> ()  [unwired: 2 in, 2 out]
                n174 = property on="Test Slider" class="Slide (strict)"("Visible"=FALSE) -> ()  [unwired: 2 in, 2 out]
              }
              frame "White Balance  **" {
                n175 = Index Array(array=w291, index=1) -> (element=w292:cluster{string[]})
                n176 = call <vilib>:"NT Read String.vi"("Name"=w294) -> ("String"=w293:string)  [unwired: 9 in, 1 out]
                n177 = Unbundle(w292) -> (w289:string[])
                n178 = Match First String(2:w289, 3:w293) -> (0:w288:i32)  [unwired: 1 out]
                n179 = property on="Test Ring" class="Ring (strict)"("Value"=w288, "Strings []"=w289) -> ()  [unwired: 2 in, 2 out]
                n180 = property on="Test Ring" class="Ring (strict)"("Visible"=TRUE) -> ()  [unwired: 2 in, 2 out]
                n181 = property on="Test Slider" class="Slide (strict)"("Visible"=FALSE) -> ()  [unwired: 2 in, 2 out]
              }
              frame "Exposure  **" {
                n182 = Index Array(array=w300, index=2) -> (element=w301:cluster{string[]})
                n183 = call <vilib>:"NT Read String.vi"("Name"=w303) -> ("String"=w302:string)  [unwired: 9 in, 1 out]
                n184 = Unbundle(w301) -> (w297:string[])
                n185 = Match First String(2:w297, 3:w302) -> (0:w298:i32)  [unwired: 1 out]
                n186 = property on="Test Ring" class="Ring (strict)"("Value"=w298, "Strings []"=w297) -> ()  [unwired: 2 in, 2 out]
                n187 = property on="Test Ring" class="Ring (strict)"("Visible"=TRUE) -> ()  [unwired: 2 in, 2 out]
                n188 = property on="Test Slider" class="Slide (strict)"("Visible"=FALSE) -> ()  [unwired: 2 in, 2 out]
              }
              frame "Exposure Priority  **" {
                n189 = Index Array(array=w309, index=3) -> (element=w310:cluster{string[]})
                n190 = call <vilib>:"NT Read String.vi"("Name"=w312) -> ("String"=w311:string)  [unwired: 9 in, 1 out]
                n191 = Unbundle(w310) -> (w306:string[])
                n192 = Match First String(2:w306, 3:w311) -> (0:w307:i32)  [unwired: 1 out]
                n193 = property on="Test Ring" class="Ring (strict)"("Value"=w307, "Strings []"=w306) -> ()  [unwired: 2 in, 2 out]
                n194 = property on="Test Ring" class="Ring (strict)"("Visible"=TRUE) -> ()  [unwired: 2 in, 2 out]
                n195 = property on="Test Slider" class="Slide (strict)"("Visible"=FALSE) -> ()  [unwired: 2 in, 2 out]
              }
              frame "Color Enable  **" {
                n196 = Index Array(array=w318, index=4) -> (element=w319:cluster{string[]})
                n197 = call <vilib>:"NT Read String.vi"("Name"=w321) -> ("String"=w320:string)  [unwired: 9 in, 1 out]
                n198 = Unbundle(w319) -> (w315:string[])
                n199 = Match First String(2:w315, 3:w320) -> (0:w316:i32)  [unwired: 1 out]
                n200 = property on="Test Ring" class="Ring (strict)"("Value"=w316, "Strings []"=w315) -> ()  [unwired: 2 in, 2 out]
                n201 = property on="Test Ring" class="Ring (strict)"("Visible"=TRUE) -> ()  [unwired: 2 in, 2 out]
                n202 = property on="Test Slider" class="Slide (strict)"("Visible"=FALSE) -> ()  [unwired: 2 in, 2 out]
              }
              frame Default {
                n203 = property on="Test Ring" class="Ring (strict)"("Visible"=FALSE) -> ()  [unwired: 2 in, 2 out]
                n204 = property on="Test Slider" class="Slide (strict)"("Visible"=FALSE) -> ()  [unwired: 2 in, 2 out]
              }
              frame "Brightness  **", "Color Level  **", "Compression  **", "FPS  **", "Sharpness  **" {
                n205 = call <vilib>:"NT Read Number.vi"("Name"=w327) -> ("Numeric"=w326:dbl)  [unwired: 9 in, 1 out]
                n206 = local write "Test Slider"(w326) -> ()
                n207 = property on="Test Slider" class="Slide (strict)"("Visible"=TRUE, "Scale.Maximum"=100.0 ("Scale.Range:Maximum")) -> ()  [unwired: 2 in, 2 out]
                n208 = property on="Test Ring" class="Ring (strict)"("Visible"=FALSE) -> ()  [unwired: 2 in, 2 out]
              }
            }
          }
        }
        n209 = property on="Progress" class="Clust (strict)"("Visible"=FALSE) -> ()  [unwired: 2 in, 2 out]
      }
      event "Test Name": Mouse Enter {
        # "Populate the ring with the list of tests"
        n210 = event-data() -> ()  [unwired: 1 in, 1 out]
        n211 = call <vilib>:"NT Read String Array.vi"("Name"="TestMode/TestList") -> ("String Array"=w335:string[])  [unwired: 9 in, 1 out]
        n212 = Build Array (concatenate)("Select the test to run...", w335) -> (w334:string[])
        n213 = property on="Test Name" class="Ring (strict)"("Strings []"=w334) -> ()  [unwired: 2 in, 2 out]
      }
      event "Test Name": Value Change {
        w337 = FALSE ("Visible")
        # "Tell the robot the test name to run"
        n214 = event-data() -> ("NewVal"=w341:u16)  [unwired: 1 in]
        n215 = property on="Test Name" class="Ring (strict)"() -> ("Strings []"=w342:string[])  [unwired: 2 in, 2 out]
        n216 = local write "Progress"(T5 {"Test Progress"=0, "Test Progress Text"=""} ("Progress")) -> ()
        n217 = Index Array(array=w342, index=w341) -> (element=w340:string)
        n218 = call <vilib>:"NT Write String.vi"("String"=w340, "Name"="TestMode/TestName") -> ()  [unwired: 9 in, 1 out]
        n219 = property on="Progress" class="Clust (strict)"("Visible"=TRUE) -> ()  [unwired: 2 in, 2 out]
        n220 = property on="Motor" class="Clust (strict)"("Visible"=w337) -> ()  [unwired: 2 in, 2 out]
        n221 = property on="Test Slider" class="Slide (strict)"("Visible"=w337) -> ()  [unwired: 2 in, 2 out]
        n222 = property on="On/Off" class="Bool (strict)"("Visible"=w337) -> ()  [unwired: 2 in, 2 out]
        n223 = property on="Rev/Fwd" class="Clust (strict)"("Visible"=w337) -> ()  [unwired: 2 in, 2 out]
        n224 = property on="Test Ring" class="Ring (strict)"("Visible"=w337) -> ()  [unwired: 2 in, 2 out]
      }
      event "Select Auto": Mouse Enter {
        # "Populate the combo box with the list of autonomous options"
        n225 = event-data() -> ()  [unwired: 1 in, 1 out]
        n226 = call <vilib>:"NT Read String Array.vi"("Name"="Auto List") -> ("String Array"=w344:string[])  [unwired: 9 in, 1 out]
        n227 = property on="Select Auto" class="CmbBox"("Strings[]"=w344) -> ()  [unwired: 2 in, 2 out]
      }
      event "Select Auto": Value Change {
        # "User modified the Auto Selection. Write to NT variable so robot knows."
        n228 = event-data() -> ("NewVal"=w347:string)  [unwired: 1 in]
        n229 = call <vilib>:"NT Write String.vi"("String"=w347, "Name"="Auto Selector") -> ()  [unwired: 9 in, 1 out]
      }
      event "Command Selection": Value Change {
        # "Get the params and show in table"
        n230 = event-data() -> ("NewVal"=w353:i32)  [unwired: 1 in]
        n231 = property on="Command Selection" class="MCListbox (strict)"() -> ("ItemNames"=w351:string[][])  [unwired: 2 in, 2 out]
        n232 = call <vilib>:"WPI_DashboardUpdate Command Params.vi"("NewVal"=w353, "Commands"=w351, "Param Tbl"=w352) -> ()  [unwired: 8 in, 1 out]
      }
      event "Execute Command": Value Change {
        # "Started one, Unique ID holds\nresponse"
        n233 = event-data() -> ()  [unwired: 1 in, 1 out]
        n234 = property on="Command Selection" class="MCListbox (strict)"() -> ("ItemNames"=w364:string[][])  [unwired: 2 in, 2 out]
        n235 = Index Array(array=w364, index (row)="Command Selection", index (col)=0) -> (element=w362:string)
        n236 = call <vilib>:"Invoke Commands.vi"("Command Params"="Command Params", "Function Name"=w362) -> ("Params"=w358:u8, "Started"=w357:bool)  [unwired: 7 in, 1 out]
        n237 = Array Subset(array="Command Params", length (row)=w358) -> (w359:string[][])  [unwired: 3 in]
        n238 = Select(t="Executing" ("Cmd Status"), s=w357, f="" ("Cmd Status")) -> (s? t:f=→"Cmd Status":string)
      }
      event "Command Selection": Double Click {
        n239 = event-data() -> ("Row"=w372:i32)  [unwired: 1 in]
        n240 = property on="Command Selection" class="MCListbox (strict)"() -> ("ItemNames"=w375:string[][])  [unwired: 2 in, 2 out]
        n241 = local read "Command Params"() -> (w371:string[][])
        n242 = Index Array(array=w375, index (row)=w372, index (col)=0) -> (element=w373:string)
        n243 = call <vilib>:"Invoke Commands.vi"("Command Params"=w371, "Function Name"=w373) -> ("Params"=w370:u8, "Started"=w365:bool)  [unwired: 7 in, 1 out]
        n244 = Array Subset(array=w371, length (row)=w370) -> (w369:string[][])  [unwired: 3 in]
        n245 = Select(t="Executing" ("Cmd Status"), s=w365, f="" ("Cmd Status")) -> (s? t:f=w366:string)
        n246 = local write "Cmd Status"(w366) -> ()
      }
      event "CheckList": Double Click {
        # "Shift clears all"
        # "Update symbols on the listbox"
        n247 = event-data() -> ("PlatMods.Shift"=w377:bool, "Row"=w379:i32)  [unwired: 1 in]
        n248 = case shown="True" w377 {
          tunnel: w379 -> [w383 _]
          tunnel: 1 -> [w382 _]
          frame False {
            n249 = property on="CheckList" class="LstBox (strict)"() -> ("Item Symbols"=w381:i32[])  [unwired: 2 in, 2 out]
            n250 = Replace Array Subset(array=w381, new element=w382, index=w383) -> (w380:i32[])
            n251 = property on="CheckList" class="LstBox (strict)"("Item Symbols"=w380) -> ()  [unwired: 2 in, 2 out]
          }
          frame True {
            w384 = 0 ("Top Row")
            n252 = property on="CheckList" class="LstBox (strict)"() -> ("Number of Rows"=w386:u32)  [unwired: 2 in, 2 out]
            n253 = Initialize Array(0, w386) -> (w385:i32[])
            n254 = property on="CheckList" class="LstBox (strict)"("Top Row"=w384, "Value"=w384, "Item Symbols"=w385) -> ()  [unwired: 2 in, 2 out]
          }
        }
      }
      event "CheckList": Key Down {
        # "Update symbols on the listbox\nLeft and right keys check and uncheck"
        n255 = event-data() -> ("VKey"=w390:T18)  [unwired: 1 in]
        n256 = case shown="\"Left\", \"Right\"" w390 {
          selector: w390 -> [w395 _]
          tunnel: eventvkey."Left" ("VKey") -> [w393 _]
          frame "Left", "Right" {
            n257 = Equal?(x=w393, y=w395) -> (x = y?=w394:bool)
            n258 = Select(t=0, s=w394, f=1) -> (s? t:f=w396:i32)
            n259 = property on="CheckList" class="LstBox (strict)"() -> ("Item Symbols"=w399:i32[])  [unwired: 2 in, 2 out]
            n260 = Replace Array Subset(array=w399, new element=w396, index="CheckList") -> (w398:i32[])
            n261 = property on="CheckList" class="LstBox (strict)"("Item Symbols"=w398) -> ()  [unwired: 2 in, 2 out]
          }
          frame Default {
          }
        }
      }
      event "Motor.Enable": Value Change {
        # "When the test mode otor enable helper is set, update that\ntree row item's value"
        n262 = event-data() -> ("NewVal"=w405:bool)  [unwired: 1 in]
        n263 = Unbundle("Motor") -> ("Value"=w404:dbl)  [unwired: 1 out]
        n264 = Select(t=w404, s=w405, f=0.0) -> (s? t:f=w402:dbl)
        n265 = call <vilib>:"NT Write Number.vi"("Numeric"=w402, "Name"=w401) -> ()  [unwired: 9 in, 1 out]
      }
      event "Test Slider": Value Change {
        # "When the test mode slider helper is set, update that\ntree row item's value"
        n266 = event-data() -> ("NewVal"=w408:dbl)  [unwired: 1 in]
        n267 = call <vilib>:"NT Write Number.vi"("Numeric"=w408, "Name"=w409) -> ()  [unwired: 9 in, 1 out]
      }
      event "On/Off": Value Change {
        # "When the test mode on/off helper value is set, update that\ntree row item's value"
        n268 = event-data() -> ("NewVal"=w413:bool)  [unwired: 1 in]
        n269 = Boolean To (0,1)(Boolean=w413) -> (0, 1=w412:i16)
        n270 = call <vilib>:"NT Write Number.vi"("Numeric"=w412, "Name"=w411) -> ()  [unwired: 9 in, 1 out]
      }
      event "Rev/Fwd": Value Change {
        # "When the test mode helper value for relays is set, update that\ntree row item's value"
        n271 = event-data() -> ("NewVal.Forward"=w421:bool, "NewVal.Reverse"=w420:bool)  [unwired: 1 in]
        n272 = Boolean To (0,1)(Boolean=w421) -> (0, 1=w417:i16)
        n273 = Boolean To (0,1)(Boolean=w420) -> (0, 1=w419:i16)
        n274 = Negate(x=w419) -> (-x=w418:i16)
        n275 = Add(x=w417, y=w418) -> (x+y=w416:i16)
        n276 = call <vilib>:"NT Write Number.vi"("Numeric"=w416, "Name"=w415) -> ()  [unwired: 9 in, 1 out]
      }
      event "Test Ring": Value Change {
        # "When a test mode helper value is selected from the ring,\nset the tree item's variable to the string value"
        n277 = event-data() -> ("NewVal"=w425:u16)  [unwired: 1 in]
        n278 = property on="Test Ring" class="Ring (strict)"() -> ("Strings []"=w426:string[])  [unwired: 2 in, 2 out]
        n279 = Index Array(array=w426, index=w425) -> (element=w424:string)
        n280 = call <vilib>:"NT Write String.vi"("String"=w424, "Name"=w423) -> ()  [unwired: 9 in, 1 out]
      }
      event "Rec Mode": Value Change {
        # "Update globals for recording mode and path to read log from.\nClear when logging and let NetworkTables set path for vision to\nuse."
        n281 = event-data() -> ("NewVal"=w437:enum32{"Stop", "Record", "Playback"})  [unwired: 1 in]
        n282 = global write "WPI_DashboardLogging Global.vi" "Logging Filename"(path "") -> ()
        n283 = global write "WPI_DashboardLogging Global.vi" "Recording"(w437) -> ()
        n284 = case shown="\"Playback\"" w437 {
          tunnel: w436 -> [_ w439 w448]
          tunnel: [_ _ w447] -> w434
          tunnel: [_ _ w446] -> _
          tunnel: w432 -> [_ _ w444]
          tunnel: cluster{i32, i32} {-250, 170} -> [_ _ w443]
          tunnel: [_ _ T19 {"Image Size"=TRUE, "Image Type"=TRUE, "Pixel Value"=TRUE, "ROI Information"=TRUE, "Zoom Factor"=FALSE} ("Image Information Shown:All Elements")] -> w427
          tunnel: [_ _ TRUE ("Zoom Factor")] -> w428
          tunnel: w430 -> [_ _ w440]
          frame Default {
          }
          frame "Stop", "Record" {
            # "Place Window too"
            n285 = invoke class="VI" method="FP.Close"(reference=w439) -> (reference out=w438:refnum<vi>)  [unwired: 2 in, 2 out]
            n286 = invoke class="VI" method="Abort VI"(reference=w438) -> ()  [unwired: 2 in, 3 out]
          }
          frame "Playback" {
            n287 = call "Open Playback Panel.vi"("Offset"=w443, "DB VI Ref"=w444, "Playback in"=w448) -> ("Playback out"=w445:refnum<vi>)  [unwired: 8 in]
            n288 = register-events(w445, w440) -> (reference out=w447:refnum<event-registration>, error out=w446:errorcluster)  [unwired: 2 in]
          }
        }
        n289 = property on="Camera Image Right" class="ImageControl"("Image Information Shown"=w427, "Image Information Visible"=w428) -> ()  [unwired: 2 in, 2 out]
        n290 = property on="Camera Image" class="ImageControl"("Image Information Shown"=w427, "Image Information Visible"=w428) -> ()  [unwired: 2 in, 2 out]
        n291 = call <vilib>:"WPI_DashboardNT Log FieldName Cache.vi"("Operation"=enum16{"Lookup/Add", "Index", "Clear"}."Clear") -> ()  [unwired: 8 in, 3 out]
      }
      event Panel Close {
        w450 = enum32{"Stop", "Record", "Playback"}."Stop" ("Rec Mode")
        # "Playback window has been closed, abort"
        n292 = event-data() -> ()  [unwired: 1 in, 4 out]
        n293 = local write "Rec Mode"(w450) -> ()
        n294 = global write "WPI_DashboardLogging Global.vi" "Recording"(w450) -> ()
      }
      event Panel Close {
        # "Abort playback window and ourself"
        n295 = event-data() -> ()  [unwired: 1 in, 4 out]
        n296 = invoke class="VI" method="FP.Close"(reference=w454) -> (reference out=w453:refnum<vi>)  [unwired: 2 in, 2 out]
        n297 = invoke class="VI" method="Abort VI"(reference=w453) -> (error out=w452:errorcluster)  [unwired: 2 in, 2 out]
        n298 = invoke class="VI" method="Abort VI"(error in=w452) -> ()  [unwired: 2 in, 3 out]
      }
      event User Event {
        n299 = event-data() -> ("IDs"=w461:cluster{"RPC field ID":u16, "Unique ID":u16}, "String"=w460:string)  [unwired: 1 in]
        n300 = Bundle("IDs"=w461, "String"=w460) -> (w459:T8)  [unwired: 1 in]
        n301 = call <vilib>:"Retrieve RPC Response.vi"("RPC Response"=w459) -> ("Output"=w457:string[][])  [unwired: 10 in]
        n302 = Build Array (concatenate)(w455, w457) -> (w456:string[][])
        n303 = local write "Command Params"(w456) -> ()
        n304 = local write "Cmd Status"("" ("Cmd Status")) -> ()
      }
      event "Tree": Double Click {
        n305 = event-data() -> ("PlatMods"=w467:T22, "Tag"=w464:string)  [unwired: 1 in]
        n306 = Unbundle(w467) -> ("Shift"=w466:bool)  [unwired: 4 out]
        n307 = String Subset(string=w464, length (rest)=1 ("length (rest)")) -> (substring=w463:string)  [unwired: 1 in]
        n308 = Not(x=w466) -> (.not. x?=w465:bool)
        n309 = case shown="\"/\"" w463 {
          tunnel: w464 -> [_ w470]
          tunnel: w465 -> [_ w469]
          frame Default {
          }
          frame "/" {
            n310 = call <vilib>:"NT Update Persistence.vi"("Persistence"=w469, "Name"=w470) -> ()  [unwired: 9 in, 1 out]
          }
        }
      }
    }
  }
  n311 = while {
    tunnel: w65 -> [w472]
    i -> [w475]
    stop <- FALSE stop-if-true
    n312 = Wait (ms)(milliseconds to wait=u32 100) -> ()  [unwired: 1 out]
    n313 = case shown="\"Playback\"" "Rec Mode" {
      tunnel: w475 -> [_ _ w490]
      tunnel: [u32 2829099 ("Base Color") u32 11141120 ("Target Color") w479] -> w471
      frame "Stop", Default {
        # "Reset the color, extra updates don't cost much"
      }
      frame "Record" {
      }
      frame "Playback" {
        # "Playback"
        n314 = Quotient & Remainder(x=w490, y=u32 50 ("milliseconds to wait")) -> (x-y*floor(x/y)=w486:u32)  [unwired: 1 out]
        n315 = Divide(x=w486, y=u32 50 ("milliseconds to wait")) -> (x/y=w483:dbl)
        n316 = Multiply(x=6.283185307179586, y=w483) -> (x*y=w488:dbl)
        n317 = Sine(x=w488) -> (sin(x)=w487:dbl)
        n318 = Absolute Value(x=w487) -> (abs(x)=w480:dbl)
        n319 = call "Interpolate RGB Color.vi"("Proportion"=w480, "Target Color"=u32 30976, "Base Color"=u32 2829099) -> ("Result Color"=w479:u32)  [unwired: 8 in]
      }
    }
    n320 = property class="Pane"(reference=w472, "PaneColor"=w471) -> ()  [unwired: 1 in, 2 out]
  }
  n321 = local write "Dashboard Tab"(T2."Drive" ("Dashboard Tab")) -> ()
  n322 = property on="On/Off" class="Bool (strict)"("Visible"=w36) -> ()  [unwired: 2 in, 2 out]
  n323 = property on="Motor" class="Clust (strict)"("Visible"=w36) -> ()  [unwired: 2 in, 2 out]
  n324 = property on="Progress" class="Clust (strict)"("Visible"=w36) -> ()  [unwired: 2 in, 2 out]
  n325 = property on="Test Ring" class="Ring (strict)"("Visible"=w36) -> ()  [unwired: 2 in, 2 out]
  n326 = property on="Rev/Fwd" class="Clust (strict)"("Visible"=w36) -> ()  [unwired: 2 in, 2 out]
  n327 = while {
    tunnel: u16 1741 ("timeout ms (25000)") -> [w492]
    stop <- FALSE stop-if-true
    n328 = TCP Create Listener(10:w492) -> (0:w491:errorcluster, 3:w493:refnum<k5>)  [unwired: 4 in, 1 out]
    n329 = case shown="No Error" w491 {
      selector: w491 -> [w495 _]
      tunnel: w493 -> [w496 _]
      frame No Error {
        n330 = while {
          tunnel: w496 -> [w499]
          tunnel: w495 -> [w498]
          stop <- FALSE stop-if-true
          n331 = TCP Wait On Listener(8:w498, 11:w499) -> (0:w500:errorcluster, 4:w501:refnum<k5>)  [unwired: 2 in, 3 out]
          n332 = local write "TCP"(w501) -> ()
          n333 = case shown="No Error" w500 {
            frame No Error {
            }
            frame Error {
              n334 = Wait (ms)(milliseconds to wait=u32 1000) -> ()  [unwired: 1 out]
            }
          }
        }
      }
      frame Error {
        n335 = Wait (ms)(milliseconds to wait=u32 1000) -> ()  [unwired: 1 out]
      }
    }
  }
  n336 = local write "Command Selection"(u16 0 ("milliseconds to wait")) -> ()
  n337 = local write "Command Params"(string[][] [] ("Command Params")) -> ()
  n338 = global write "WPI_DashboardLogging Global.vi" "Recording"(w59) -> ()
  n339 = local write "Rec Mode"(w59) -> ()
  n340 = call <vilib>:"NT Write String.vi"("String"="Select Auto", "Name"="Auto Selector") -> ()  [unwired: 9 in, 1 out]
